vi "loadUpChannels.vi"(8 "error in (no error)":errorcluster, 10 "ChannelArray":refnum<class "ChannelArray.lvclass">, 11 "ScriptEventList in":refnum<class "ScriptEventList.lvclass">) -> (0 "error out":errorcluster, 3 "ScriptEventList out":refnum<class "ScriptEventList.lvclass">)   [LabVIEW 2009, in "Tools.lvlib" / "Scripting.lvlib" / "ScriptEventList.lvclass"]
uses:
  ScriptEventList.lvclass
  DatabaseHelpers/Database Objects/ChannelArray/ChannelArray.lvclass
  ScriptEventList.lvclass/ScriptEventList.ctl
  ScriptEvent.lvclass
  DatabaseHelpers/Database Objects/Channel/Channel.lvclass
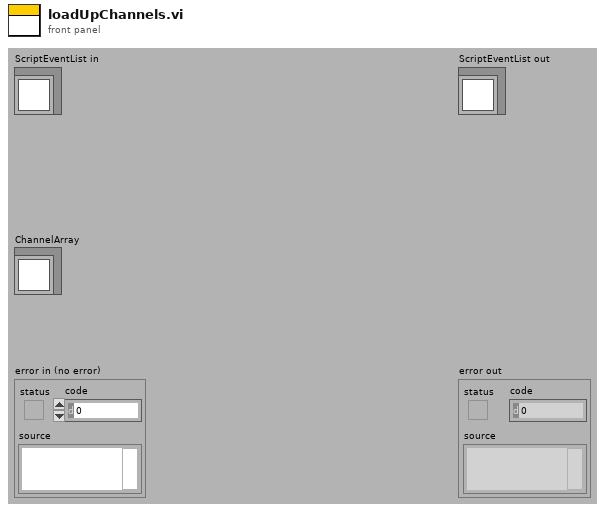
[diagram p1: front panel]
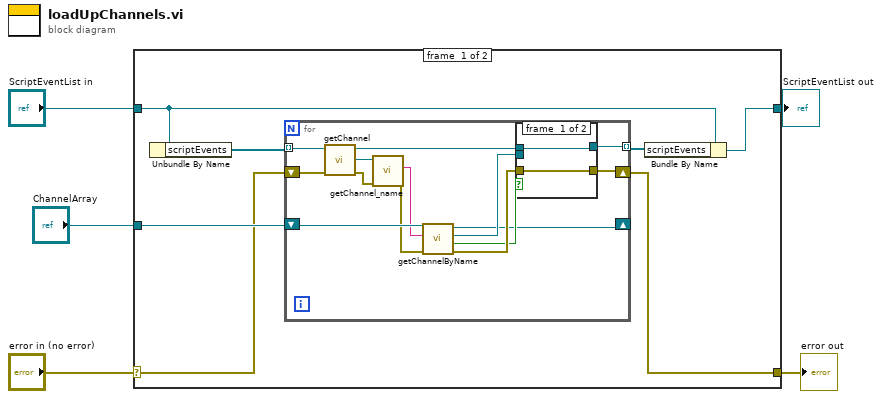
[diagram p0: block diagram]
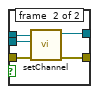
[diagram p2: hidden frame]
diagram:
  n1 = case shown="No Error" "error in (no error)" {
    selector: "error in (no error)" -> [w10 w35]
    tunnel: [w6 w35] -> w4
    tunnel: [w7 w34] -> w2
    tunnel: "ScriptEventList in" -> [w8 w34]
    tunnel: "ChannelArray" -> [w11 _]
    frame #0 {
      n2 = Unbundle By Name(w8) -> ("scriptEvents"=w12:refnum<class "ScriptEvent.lvclass">[])
      n3 = for {
        tunnel: w12 -> [w25] mode=indexing
        shift-right: [w15] -> w6
        shift-left: w10 -> [w18]
        shift-right: [w14] -> _
        shift-left: w11 -> [w26]
        tunnel: [w13] -> w9 mode=indexing
        n4 = call-dynamic "getChannel.vi"("error in (no error)"=w18, "ScriptEvent.lvclass in"=w25) -> ("error out"=w24:errorcluster, "Channel.lvclass"=w23:refnum<class "Channel.lvclass">, "ScriptEvent.lvclass out"=w22:refnum<class "ScriptEvent.lvclass">)  [unwired: 7 in]
        n5 = call "getChannel_name.vi"("error in (no error)"=w24, "Channel.lvclass in"=w23) -> ("error out"=w19:errorcluster, "channel_name"=w20:string)  [unwired: 7 in, 1 out]
        n6 = call-dynamic "getChannelByName.vi"("error in (no error)"=w19, "channel_name"=w20, "ChannelArray in"=w26) -> ("error out"=w17:errorcluster, "found?"=w16:bool, "Channel"=w21:refnum<class "Channel.lvclass">, "ChannelArray out"=w14:refnum<class "ChannelArray.lvclass">)  [unwired: 5 in]
        n7 = case shown="True" w16 {
          tunnel: w22 -> [w28 w33]
          tunnel: w21 -> [_ w32]
          tunnel: w17 -> [w27 w31]
          tunnel: [w28 w30] -> w13
          tunnel: [w27 w29] -> w15
          frame #0 {
          }
          frame #1 {
            n8 = call-dynamic "setChannel.vi"("error in (no error)"=w31, "Channel.lvclass"=w32, "ScriptEvent.lvclass in"=w33) -> ("error out"=w29:errorcluster, "ScriptEvent.lvclass out"=w30:refnum<class "ScriptEvent.lvclass">)  [unwired: 7 in]
          }
        }
      }
      n9 = Bundle By Name(cluster=w8, "scriptEvents"=w9) -> (w7:refnum<class "ScriptEventList.lvclass">)
    }
    frame #1 {
    }
  }
  "error out" <- w4
  "ScriptEventList out" <- w2
